vi "Measurement Logic.vi"() -> ()   [LabVIEW 2024, in "PMIC_Efficiency_DMM.lvlib"]
uses:
  PMIC_Efficiency_DMM.lvlib
  Measurement Configuration.ctl
  measurementlink-labview-examples-2.0.0.1/NI-DMM Measurement/NIDmmMeasurement/ResolutionInDigits.ctl
  Measurement Results.ctl
  <vilib>/gRPC/Generated APIs/ni/protobuf/types/RPC Messages/ni_protobuf_types_DoubleXYData.ctl
  <vilib>/MeasurementLink/MeasurementLink Measurement Server/Measure Call Context/Measure Call Context.lvclass
  <vilib>/MeasurementLink/MeasurementLink Measurement Server/Measure Call Context/Reserve Sessions - NPin.vi
  <vilib>/MeasurementLink/MeasurementLink niDCPower/Initialize Sessions - NSess.vi
  <vilib>/MeasurementLink/MeasurementLink niDCPower/Get Connections - NPin MConn.vi
  <vilib>/MeasurementLink/MeasurementLink niDMM/Initialize Sessions - 1Sess.vi
  <vilib>/MeasurementLink/MeasurementLink niDMM/Get Connections - 1Pin 1Conn.vi
  <vilib>/MeasurementLink/MeasurementLink niDCPower/MeasurementLink niDCPower.lvlib
  <vilib>/MeasurementLink/MeasurementLink Session Management V1/Session Reservation/Session Reservation.lvclass
  <vilib>/MeasurementLink/MeasurementLink niDMM/MeasurementLink niDMM.lvlib
  measurementlink-labview-examples-2.0.0.1/NI-DMM Measurement/NIDmmMeasurement/NIDmmMeasurement.lvlib
  <vilib>/gRPC/Generated APIs/ni/protobuf/types/ni.protobuf.types.lvlib
panel:
  out "measure call context out":refnum<class "Measure Call Context.lvclass">
  in  "measure call context in":refnum<class "Measure Call Context.lvclass">
  out "measurement results":T1
  in  "measurement configuration":T3={"Vin Pin Name"="", "Source Voltage Level (V)"=3.0, "Source Current Limit (A)"=1.0, "Eload Pin Name"="", "Load Voltage Limit (V)"=5.0, "Points"=10, "Current Load Level Start"=0.1, "Current Load Level Stop"=1.0, "Vout Pin Name"="", "Range"=10.0, "Resolution in Digits"=enum."5 1/2"} {"Range" min=0.0 step=0.1; "Current Load Level Stop" min=1.0; "Points" min=1; "Source Current Limit (A)" format="%#_6p"; "Source Voltage Level (V)" format="%#_6p"}
  out "error out":errorcluster
  in  "error in":errorcluster
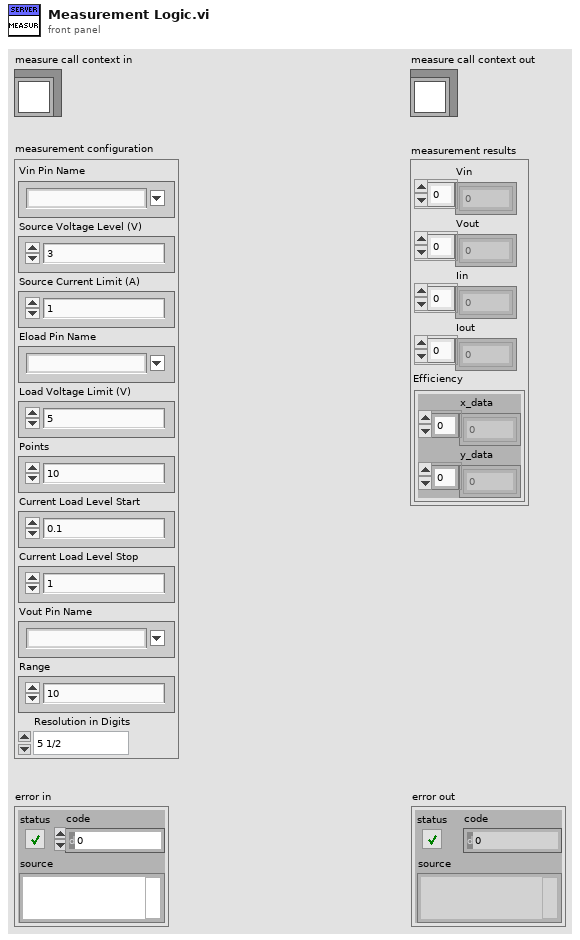
[diagram p1: front panel]
types:
  T1 = typedef "PMIC_Efficiency_DMM.lvlib/Measurement Results.ctl" = cluster{"Vin":dbl[], "Vout":dbl[], "Iin":dbl[], "Iout":dbl[], "Efficiency":T2}
  T2 = typedef "ni.protobuf.types.lvlib/ni_protobuf_types_DoubleXYData.ctl" = cluster{"x_data":dbl[], "y_data":dbl[]}
  T3 = typedef "PMIC_Efficiency_DMM.lvlib/Measurement Configuration.ctl" = cluster{"Vin Pin Name":string, "Source Voltage Level (V)":dbl, "Source Current Limit (A)":dbl, "Eload Pin Name":string, "Load Voltage Limit (V)":dbl, "Points":i32, "Current Load Level Start":dbl, "Current Load Level Stop":dbl, "Vout Pin Name":string, "Range":dbl, "Resolution in Digits":T4}
  T4 = typedef "NIDmmMeasurement.lvlib/ResolutionInDigits.ctl" = enum32{"3 1/2", "4 1/2", "5 1/2", "6 1/2", "7 1/2"}
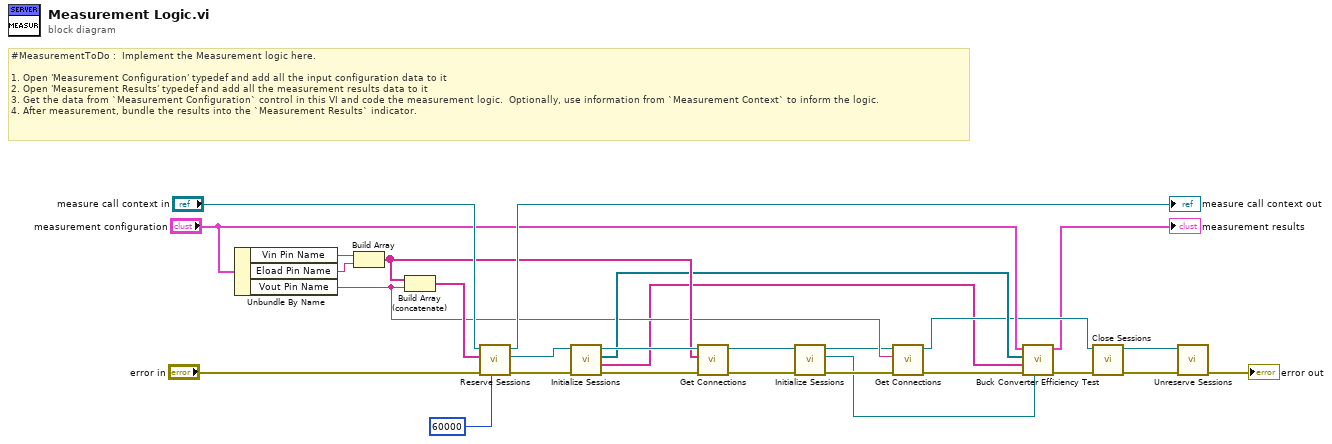
[diagram p0: block diagram]
diagram:
  # "#MeasurementToDo :  Implement the Measurement logic here.\n\n1. Open 'Measurement Configuration' typedef and add all the input configuration data to it\n2. Open 'Measurement Results' typedef and add all the measurement results data to it\n3. Get the data from `Measurement Configuration` control in this VI and code the measurement logic.  Optionally, use information from `Measurement Context` to inform the logic.\n4. After measurement, bundle the results into the `Measurement Results` indicator."
  n1 = Unbundle By Name("measurement configuration") -> ("Vin Pin Name"=w14:string, "Eload Pin Name"=w21:string, "Vout Pin Name"=w8:string)
  n2 = Build Array(w14, w21) -> (w13:string[])
  n3 = Build Array (concatenate)(w13, w8) -> (w12:string[])
  n4 = call-poly <vilib>:"Reserve Sessions.vi"("timeout (ms)"=60000, "error in"="error in", "pin or relay names"=w12, "measurement context in"="measure call context in") -> ("error out"=w15:errorcluster, "session reservation out"=w16:refnum<class "Session Reservation.lvclass">, "measurement context out"=→"measure call context out":refnum<class "Measure Call Context.lvclass">)  [unwired: 5 in]
  n5 = call-poly <vilib>:"Initialize Sessions.vi"("error in"=w15, "session reservation in"=w16) -> ("error out"=w18:errorcluster, "channel lists"=w3:string[], "sessions"=w11:refnum<k15>[], "session reservation out"=w17:refnum<class "Session Reservation.lvclass">)  [unwired: 6 in]
  n6 = call-poly <vilib>:"Get Connections.vi"("error in"=w18, "pin or relay names"=w13, "session reservation in"=w17) -> ("error out"=w9:errorcluster, "session reservation out"=w10:refnum<class "Session Reservation.lvclass">)  [unwired: 6 in, 1 out]
  n7 = call-poly <vilib>:"Initialize Sessions.vi"("error in"=w9, "session reservation in"=w10) -> ("error out"=w6:errorcluster, "session"=w2:refnum<k15>, "session reservation out"=w7:refnum<class "Session Reservation.lvclass">)  [unwired: 6 in, 1 out]
  n8 = call-poly <vilib>:"Get Connections.vi"("error in"=w6, "pin or relay name"=w8, "session reservation in"=w7) -> ("error out"=w5:errorcluster, "session reservation out"=w4:refnum<class "Session Reservation.lvclass">)  [unwired: 6 in, 1 out]
  n9 = call "Buck Converter Efficiency Test.vi"("DMM Session"=w2, "error in (no error)"=w5, "Channel List"=w3, "DCPower Session"=w11, "measurement configuration"="measurement configuration") -> ("error out"=w20:errorcluster, "measurement results"=→"measurement results":T1)  [unwired: 5 in]
  n10 = call <vilib>:"Close Sessions.vi"("error in"=w20, "session reservation in"=w4) -> ("error out"=w23:errorcluster, "session reservation out"=w24:refnum<class "Session Reservation.lvclass">)  [unwired: 8 in]
  n11 = call <vilib>:"Unreserve Sessions.vi"("error in"=w23, "session reservation in"=w24) -> ("error out"=→"error out":errorcluster)  [unwired: 9 in]
